vi "Create Paragraph Collection.vi"(8 "error in (no error)":errorcluster, 10 "Text":string, 11 "ooWriter in":refnum<class "ooCalc.lvclass">) -> (0 "error out":errorcluster, 2 "Paragraph Collection":refnum<k24>, 3 "ooWriter out":refnum<class "ooCalc.lvclass">)   [LabVIEW 2009, in "ooCalc.lvclass"]
uses:
  ooCalc.lvclass
  C:/Projets/LAVAG/OpenOfficeRGT/AODL/DLLs/AODL.dll
  ooCalc.lvclass/ooCalc.ctl
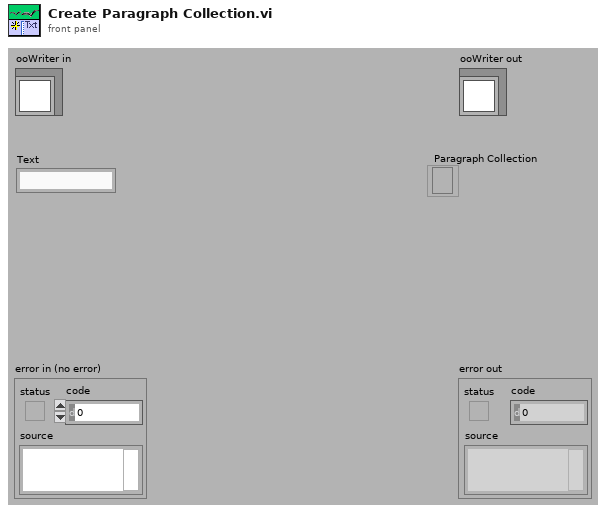
[diagram p1: front panel]
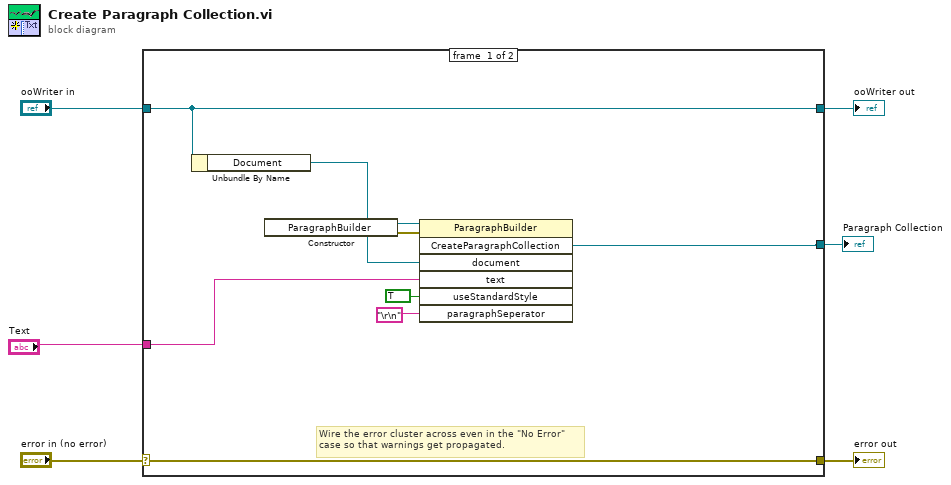
[diagram p0: block diagram]
diagram:
  n1 = case shown="No Error" "error in (no error)" {
    selector: "error in (no error)" -> [w15 w17]
    tunnel: [w15 w17] -> w5
    tunnel: [w12 w16] -> w3
    tunnel: "ooWriter in" -> [w12 w16]
    tunnel: "Text" -> [w10 _]
    tunnel: [w7 _] -> w1
    frame #0 {
      # "Wire the error cluster across even in the \"No Error\"\ncase so that warnings get propagated."
      n2 = Unbundle By Name(w12) -> ("Document"=w11:refnum<k24>)
      n3 = constructor class="ParagraphBuilder"() -> (reference out=w13:refnum<k24>, error out=w14:errorcluster)  [unwired: 3 in, 1 out]
      n4 = invoke class="ParagraphBuilder" method="CreateParagraphCollection"(reference=w13, error in=w14, "document"=w11, "text"=w10, "useStandardStyle"=TRUE, "paragraphSeperator"="\r\n") -> ("CreateParagraphCollection"=w7:refnum<k24>)  [unwired: 1 in, 6 out]
    }
    frame #1 {
    }
  }
  "error out" <- w5
  "ooWriter out" <- w3
  "Paragraph Collection" <- w1
